vi "Contains Key.vi"(10 "Key":string, 11 "Section in":refnum<class "Section.lvclass">) -> (1 "Contains Key?":bool, 2 "Index":i32, 3 "Section out":refnum<class "Section.lvclass">)   [LabVIEW 2024, in "Electronic Datasheet.lvlib" / "Section.lvclass"]
uses:
  Section.lvclass
  Section.lvclass/Section.ctl
  Keyname/Key Name.lvclass
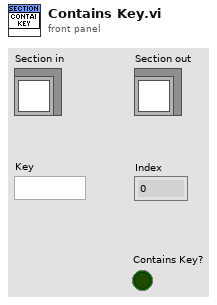
[diagram p1: front panel]
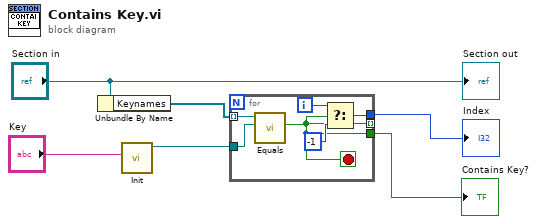
[diagram p0: block diagram]
diagram:
  n1 = Unbundle By Name("Section in") -> ("Keynames"=w5:refnum<class "Key Name.lvclass">[])
  n2 = call "Init.vi"("Key Name"="Key") -> ("Key Name out"=w3:refnum<class "Key Name.lvclass">)  [unwired: 9 in, 1 out]
  n3 = for {
    tunnel: w5 -> [w12] mode=indexing
    tunnel: [w9] -> w1 if=w7
    tunnel: w3 -> [w11]
    tunnel: [w7] -> _ mode=indexing
    tunnel: [w7] -> w2
    i -> [w10]
    stop <- w7 stop-if-true
    n4 = call "Equals.vi"("Keyname"=w11, "Keyname in"=w12) -> ("Equal?"=w7:bool)  [unwired: 8 in, 1 out]
    n5 = Select(t=w10, s=w7, f=-1) -> (s? t:f=w9:i32)
  }
  "Contains Key?" <- w2
  "Index" <- w1
  "Section out" <- "Section in"
